vi "Error Query.vi"(0 "VISA resource name":refnum<visa-resource-name>, 11 "error in (no error)":errorcluster) -> (4 "VISA resource name out":refnum<visa-resource-name>, 8 "Error":i32, 10 "Error Message":string, 15 "error out":errorcluster)   [LabVIEW 2013, in "Yokogawa WT200 Series.lvlib"]
doc: "This VI reads an error from the instrument. It expects to see errors in SCPI format (#,\"error message\")."
uses:
  <instrlib>/Yokogawa WT200 Series/Yokogawa WT200 Series.lvlib
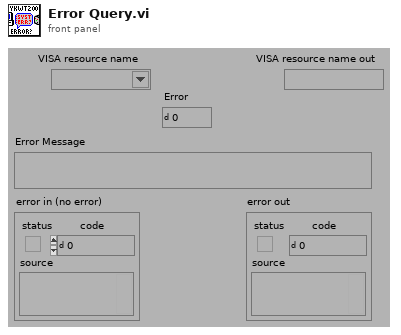
[diagram p1: front panel]
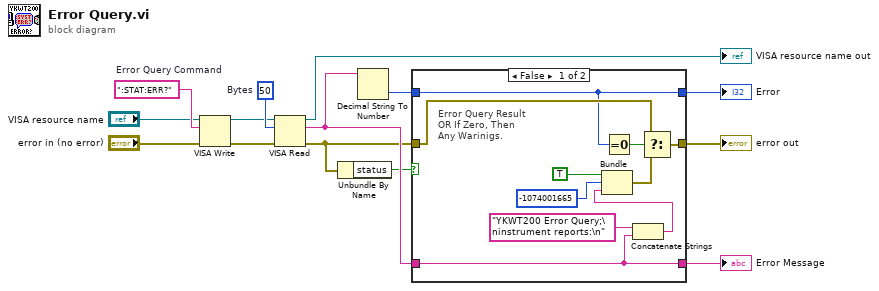
[diagram p0: block diagram]
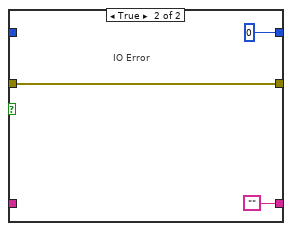
[diagram p2: hidden frame]
diagram:
  w9 = u32 50  # Bytes
  w11 = ":STAT:ERR?"  # Error Query Command
  n1 = VISA Write(VISA resource name="VISA resource name", write buffer=w11, error in (no error)="error in (no error)") -> (VISA resource name out=w8:refnum<visa-resource-name>, error out=w10:errorcluster)  [unwired: 1 out]
  n2 = VISA Read(VISA resource name=w8, byte count=w9, error in (no error)=w10) -> (VISA resource name out=→"VISA resource name out":refnum<visa-resource-name>, read buffer=w13:string, error out=w7:errorcluster)  [unwired: 1 out]
  n3 = Unbundle By Name(w7) -> ("status"=w12:bool)
  n4 = Decimal String To Number(string=w13) -> (number=w14:i32)  [unwired: 2 in, 1 out]
  n5 = case shown="False" w12 {
    tunnel: w13 -> [w22 _]
    tunnel: w7 -> [w18 w27]
    tunnel: [w19 w27] -> w2
    tunnel: [w22 ""] -> w1
    tunnel: [w15 0] -> w3
    tunnel: w14 -> [w15 _]
    frame False {
      # "Error Query Result\nOR If Zero, Then\nAny Warinigs."
      n6 = Equal To 0?(x=w15) -> (x = 0?=w16:bool)
      n7 = Concatenate Strings("YKWT200 Error Query;\ninstrument reports:\n" ("Source"), w22) -> (w21:string)
      n8 = Bundle("Status"=TRUE, "Code"=-1074001665, w21) -> (w20:cluster{"Status":bool, "Code":i32, string})  [unwired: 1 in]
      n9 = Select(t=w18, s=w16, f=w20) -> (s? t:f=w19:errorcluster)
    }
    frame True {
      # "IO Error"
    }
  }
  "Error Message" <- w1
  "Error" <- w3
  "error out" <- w2
